vi "Symbol_File_Parser.vi"(8 "error in (no error)":errorcluster, 11 "Symbol File Path":path) -> (0 "error out":errorcluster, 2 "Parameters":T6[](array[typedef]), 3 "Data Packets":T1[](array[typedef]))   [LabVIEW 2017]
uses:
  Controls/Data Packets/Parameter.ctl
  Controls/Data Packets/Parameter_Data_Type.ctl
  Controls/Data Packets/Data_Packet.ctl
  Controls/Packet/Packet.ctl
  Controls/Packet/Packet_Direction.ctl
  Controls/Packet/Packet_Type.ctl
  Controls/Packet/Packet_Priority.ctl
  Controls/Data Packets/Data_Packet_Transmit_Mode.ctl
  <vilib>/Utility/file.llb/Read Delimited Spreadsheet (string).vi
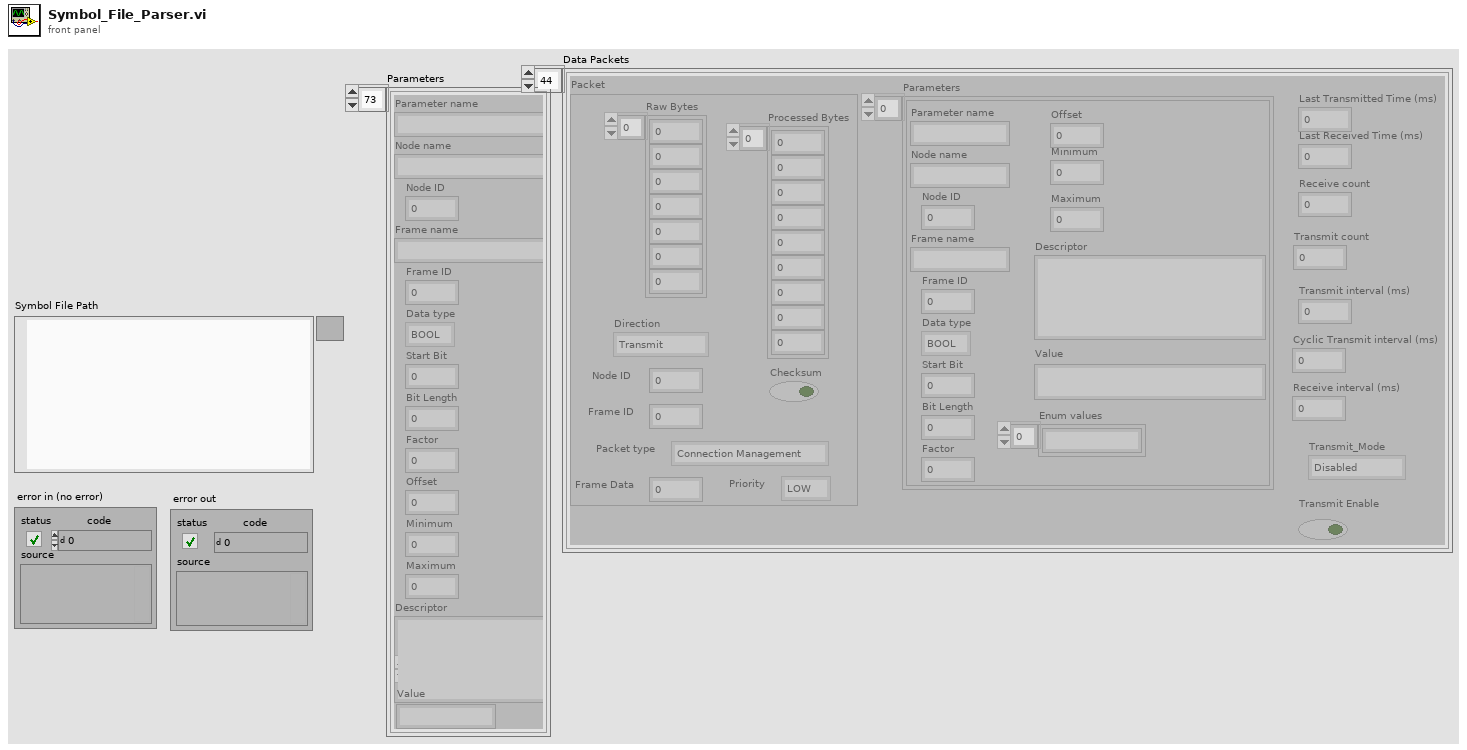
[diagram p1: front panel]
types:
  T1 = typedef "Data_Packet.ctl" = cluster{"Packet":T2, "Parameters":T6[], "Last Received Time (ms)":u64, "Receive count":i32, "Transmit count":i32, "Transmit interval (ms)":u32, "Last Transmitted Time (ms)":u64, "Receive interval (ms)":u32, "Transmit_Mode":T8, "Transmit Enable":bool, "Cyclic Transmit interval (ms)":u32}
  T2 = typedef "Packet.ctl" = cluster{"Raw Bytes":u8[], "Checksum":bool, "Direction":T3, "Processed Bytes":u8[], "Node ID":u8, "Packet type":T4, "Frame Data":u32, "Priority":T5, "Frame ID":u8}
  T3 = typedef "Packet_Direction.ctl" = enum16{"Transmit", "Receive", "Bidirectional"}
  T4 = typedef "Packet_Type.ctl" = enum16{"Data", "Connection Management", "Remote Request", "Error/Status"}
  T5 = typedef "Packet_Priority.ctl" = enum16{"LOW", "HIGH"}
  T6 = typedef "Parameter.ctl" = cluster{"Parameter name":string, "Node name":string, "Node ID":u8, "Frame name":string, "Frame ID":u8, "Data type":T7, "Start Bit":i32, "Bit Length":i32, "Factor":dbl, "Offset":dbl, "Minimum":dbl, "Maximum":dbl, "Descriptor":string, "Enum values":string[], "Value":string}
  T7 = typedef "Parameter_Data_Type.ctl" = enum16{"BOOL", "UNSIGNED", "SIGNED", "FLOAT32", "ENUM"}
  T8 = typedef "Data_Packet_Transmit_Mode.ctl" = enum16{"Disabled", "Single", "Cyclic"}
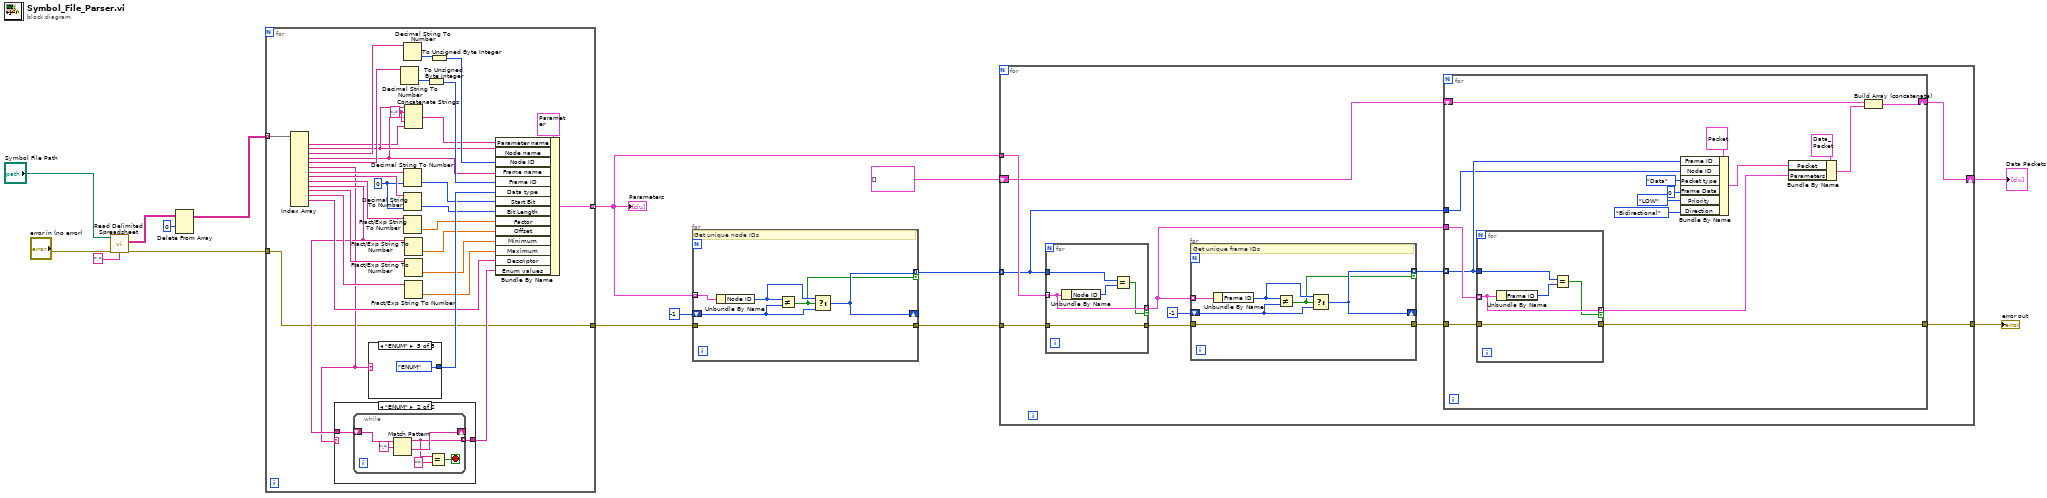
[diagram p0: block diagram]
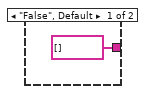
[diagram p2: hidden frame]
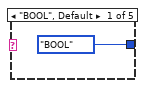
[diagram p3: hidden frame]
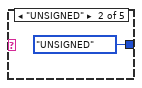
[diagram p4: hidden frame]
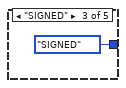
[diagram p5: hidden frame]
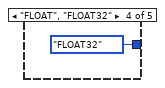
[diagram p6: hidden frame]
diagram:
  n1 = call-poly <vilib>:"Read Delimited Spreadsheet.vi"("file path (dialog if empty)"="Symbol File Path", "error in (no error)"="error in (no error)", "delimiter (\\t)"="," ("delimiter (\\t)")) -> ("all rows"=w3:string[][], "error out"=w13:errorcluster)  [unwired: 7 in, 4 out]
  n2 = Delete From Array(array=w3, index (row)=0) -> (array with subset deleted=w2:string[][])  [unwired: 2 in, 1 out]
  n3 = for {
    tunnel: w13 -> [w21]
    tunnel: w2 -> [w46] mode=indexing
    tunnel: [w25] -> w7 mode=indexing
    tunnel: [w21] -> w10
    w20 = ":" ("string")
    w36 = u8 0 ("default (0 I32)")
    n4 = Index Array(array=w46) -> (element #1=w16:string, element #2=w18:string, element #3=w45:string, element #4=w17:string, element #5=w41:string, element #6=w22:string, element #7=w38:string, element #8=w37:string, element #9=w33:string, element #10=w23:string, element #11=w30:string, element #12=w29:string, element #13=w26:string)  [unwired: 14 in, 1 out]
    n5 = case shown="\"ENUM\"" w22 {
      tunnel: [string[] [] w50] -> w24
      tunnel: w23 -> [_ w49]
      frame "False", Default {
      }
      frame "ENUM" {
        n6 = while {
          shift-right: [w55] -> _
          shift-left: w49 -> [w56]
          tunnel: [w51] -> w50 mode=indexing
          stop <- w53 stop-if-true
          n7 = Match Pattern(string=w56, regular expression=":") -> (before substring=w51:string, after substring=w55:string)  [unwired: 1 in, 2 out]
          n8 = Equal?(x=w51, y="") -> (x = y?=w53:bool)
        }
      }
    }
    n9 = case shown="\"ENUM\"" w22 {
      tunnel: [Parameter_Data_Type."BOOL" ("Data type") Parameter_Data_Type."UNSIGNED" ("Data type") Parameter_Data_Type."SIGNED" ("Data type") Parameter_Data_Type."FLOAT32" ("Data type") Parameter_Data_Type."ENUM" ("Data type")] -> w39
      frame "BOOL", Default {
      }
      frame "UNSIGNED" {
      }
      frame "SIGNED" {
      }
      frame "FLOAT", "FLOAT32" {
      }
      frame "ENUM" {
      }
    }
    n10 = Decimal String To Number(string=w41) -> (number=w42:i32)  [unwired: 2 in, 1 out]
    n11 = Decimal String To Number(string=w45) -> (number=w44:i32)  [unwired: 2 in, 1 out]
    n12 = Decimal String To Number(string=w38, default (0L)=w36) -> (number=w35:u8)  [unwired: 1 in, 1 out]
    n13 = Decimal String To Number(string=w37, default (0L)=w36) -> (number=w34:u8)  [unwired: 1 in, 1 out]
    n14 = Fract/Exp String To Number(string=w33) -> (number=w32:dbl)  [unwired: 3 in, 1 out]
    n15 = Concatenate Strings(w18, w20, w17, w20, w16) -> (w19:string)
    n16 = Fract/Exp String To Number(string=w23) -> (number=w31:dbl)  [unwired: 3 in, 1 out]
    n17 = Fract/Exp String To Number(string=w29) -> (number=w27:dbl)  [unwired: 3 in, 1 out]
    n18 = Fract/Exp String To Number(string=w30) -> (number=w28:dbl)  [unwired: 3 in, 1 out]
    n19 = To Unsigned Byte Integer(number=w42) -> (unsigned 8bit integer=w40:u8)
    n20 = To Unsigned Byte Integer(number=w44) -> (unsigned 8bit integer=w43:u8)
    n21 = Bundle By Name(cluster=T6 {"Parameter name"="", "Node name"="", "Node ID"=0, "Frame name"="", "Frame ID"=0, "Data type"=enum."BOOL", "Start Bit"=0, "Bit Length"=0, "Factor"=0.0, "Offset"=0.0, "Minimum"=0.0, "Maximum"=0.0, "Descriptor"="", "Enum values"=[], "Value"=""} ("Parameter"), "Parameter name"=w19, "Node name"=w18, "Node ID"=w43, "Frame name"=w17, "Frame ID"=w40, "Data type"=w39, "Start Bit"=w35, "Bit Length"=w34, "Factor"=w32, "Offset"=w31, "Minimum"=w28, "Maximum"=w27, "Descriptor"=w26, "Enum values"=w24) -> (w25:T6)
  }
  "Parameters" <- w7
  n22 = for {
    tunnel: w10 -> [w62]
    shift-right: [w64] -> _
    shift-left: -1 -> [w67]
    tunnel: w7 -> [w66] mode=indexing
    tunnel: [w64] -> w9 mode=indexing if=w63
    tunnel: [w62] -> w8
    # "Get unique node IDs"
    n23 = Unbundle By Name(w66) -> ("Node ID"=w65:u8)
    n24 = Not Equal?(x=w65, y=w67) -> (x != y?=w63:bool)
    n25 = Select(t=w65, s=w63, f=w67) -> (s? t:f=w64:i32)
  }
  n26 = for {
    tunnel: w9 -> [w72] mode=indexing
    tunnel: w8 -> [w78]
    tunnel: w7 -> [w77]
    shift-right: [w69] -> w5
    shift-left: T1[] [] -> [w70]
    tunnel: [w68] -> w4
    n27 = for {
      tunnel: w78 -> [w106]
      tunnel: w77 -> [w108] mode=indexing
      tunnel: w72 -> [w109]
      tunnel: [w108] -> w71 mode=indexing if=w107
      tunnel: [w106] -> w75
      n28 = Unbundle By Name(w108) -> ("Node ID"=w110:u8)
      n29 = Equal?(x=w109, y=w110) -> (x = y?=w107:bool)
    }
    n30 = for {
      tunnel: w75 -> [w100]
      shift-right: [w102] -> _
      shift-left: -1 -> [w105]
      tunnel: w71 -> [w104] mode=indexing
      tunnel: [w102] -> w73 mode=indexing if=w101
      tunnel: [w100] -> w74
      # "Get unique frame IDs"
      n31 = Unbundle By Name(w104) -> ("Frame ID"=w103:u8)
      n32 = Not Equal?(x=w103, y=w105) -> (x != y?=w101:bool)
      n33 = Select(t=w103, s=w101, f=w105) -> (s? t:f=w102:i32)
    }
    n34 = for {
      tunnel: w74 -> [w93]
      tunnel: w73 -> [w89] mode=indexing
      tunnel: w72 -> [w88]
      tunnel: w71 -> [w94]
      shift-right: [w80] -> w69
      shift-left: w70 -> [w82]
      tunnel: [w79] -> w68
      n35 = for {
        tunnel: w94 -> [w97] mode=indexing
        tunnel: w89 -> [w99]
        tunnel: [w97] -> w91 mode=indexing if=w96
        tunnel: w93 -> [w95]
        tunnel: [w95] -> w79
        n36 = Unbundle By Name(w97) -> ("Frame ID"=w98:u8)
        n37 = Equal?(x=w99, y=w98) -> (x = y?=w96:bool)
      }
      n38 = Bundle By Name(cluster=T2 {"Raw Bytes"=[], "Checksum"=FALSE, "Direction"=enum."Transmit", "Processed Bytes"=[], "Node ID"=0, "Packet type"=enum."Connection Management", "Frame Data"=0, "Priority"=enum."LOW", "Frame ID"=0} ("Packet"), "Frame ID"=w89, "Node ID"=w88, "Packet type"=Packet_Type."Data", "Frame Data"=u32 0, "Priority"=Packet_Priority."LOW", "Direction"=Packet_Direction."Bidirectional") -> (w83:T2)
      n39 = Bundle By Name(cluster=T1 {"Packet"={"Raw Bytes"=[], "Checksum"=FALSE, "Direction"=enum."Transmit", "Processed Bytes"=[], "Node ID"=0, "Packet type"=enum."Connection Management", "Frame Data"=0, "Priority"=enum."LOW", "Frame ID"=0}, "Parameters"=[], "Last Received Time (ms)"=0, "Receive count"=0, "Transmit count"=0, "Transmit interval (ms)"=0, "Last Transmitted Time (ms)"=0, "Receive interval (ms)"=0, "Transmit_Mode"=enum."Disabled", "Transmit Enable"=FALSE, "Cyclic Transmit interval (ms)"=0} ("Data_Packet"), "Packet"=w83, "Parameters"=w91) -> (w81:T1)
      n40 = Build Array (concatenate)(w82, w81) -> (w80:T1[])
    }
  }
  "error out" <- w4
  "Data Packets" <- w5
